vi "Get BrowerComponents.vi"(8 "error in (no error)":errorcluster, 11 "BrowerComposite in":refnum<class "BrowerComposite.lvclass">) -> (0 "error out":errorcluster, 2 "BrowerComponents":refnum<class "BrowerComponent.lvclass">[](array[class]), 3 "BrowerComposite out":refnum<class "BrowerComposite.lvclass">)   [LabVIEW 2015, in "BrowerComposite.lvclass"]
uses:
  BrowerComposite.lvclass
  BrowerComponent/BrowerComponent.lvclass
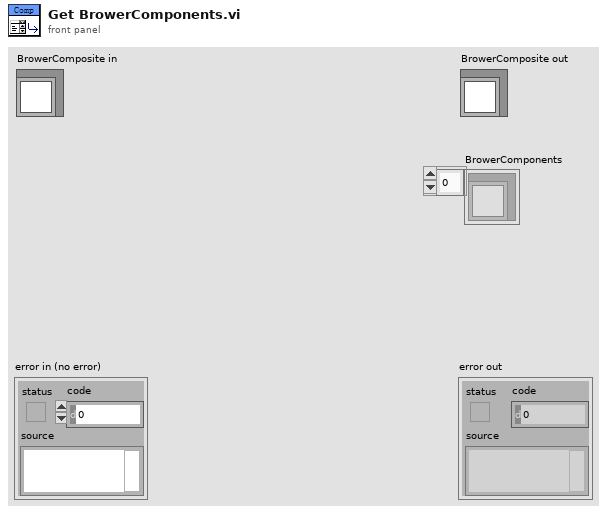
[diagram p1: front panel]
types:
  T1 = typedef "BrowerComposite.lvclass/ObjectAttributes.ctl" = cluster{"BrowerComponents":refnum<class "BrowerComponent.lvclass">[], "BrowerComponentIDs":string[], "Iterator":refnum<class "Iterator.lvclass">}
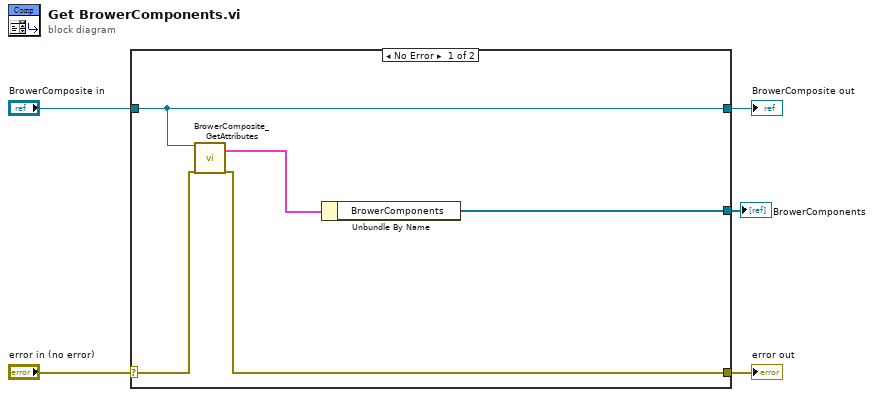
[diagram p0: block diagram]
diagram:
  n1 = case shown="No Error" "error in (no error)" {
    selector: "error in (no error)" -> [w9 w12]
    tunnel: [w8 w12] -> w4
    tunnel: [w10 w11] -> w2
    tunnel: "BrowerComposite in" -> [w10 w11]
    tunnel: [w6 _] -> w1
    frame No Error {
      n2 = call "BrowerComposite_GetAttributes.vi"("reference in"=w10, "error in (no error)"=w9) -> ("Data"=w7:T1, "error out"=w8:errorcluster)  [unwired: 14 in, 2 out]
      n3 = Unbundle By Name(w7) -> ("BrowerComponents"=w6:refnum<class "BrowerComponent.lvclass">[])
    }
    frame Error {
    }
  }
  "error out" <- w4
  "BrowerComposite out" <- w2
  "BrowerComponents" <- w1
